vi "Match.vi"   [LabVIEW 2020, in "Stream.lvlib" / "URLPattern.lvclass"]
uses:
  URLPattern.lvclass
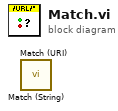
[diagram p0: block diagram]
diagram:
  n1 = call "Match (String).vi"() -> ()  [unwired: 8 in, 4 out]
  n2 = call "Match (URI).vi"() -> ()  [unwired: 8 in, 4 out]
